vi "Biometry Average Ascan Parameter2String.vi"(8 "error in (no error)":errorcluster caption="错误输入（无错误）", 9 "Biometry Average Standard Deviation":T1, 10 "Biometry Average State":T2, 11 "Biometry Average Parameter":T3) -> (0 "error out":errorcluster caption="错误输出", 2 "Data Output":string[][](array[string]))   [LabVIEW 2015, in "Utility VIs.lvlib"]
doc: "该模板用于创建子VI。"
uses:
  Utility VIs.lvlib
  Database Processing/Support/Table/Biometry Average Parameter.ctl
  Database Processing/Support/Table/Biometry Average State.ctl
  Database Processing/Support/Table/Biometry Average Standard Deviation.ctl
  Database Processing/Database Processing.lvlib
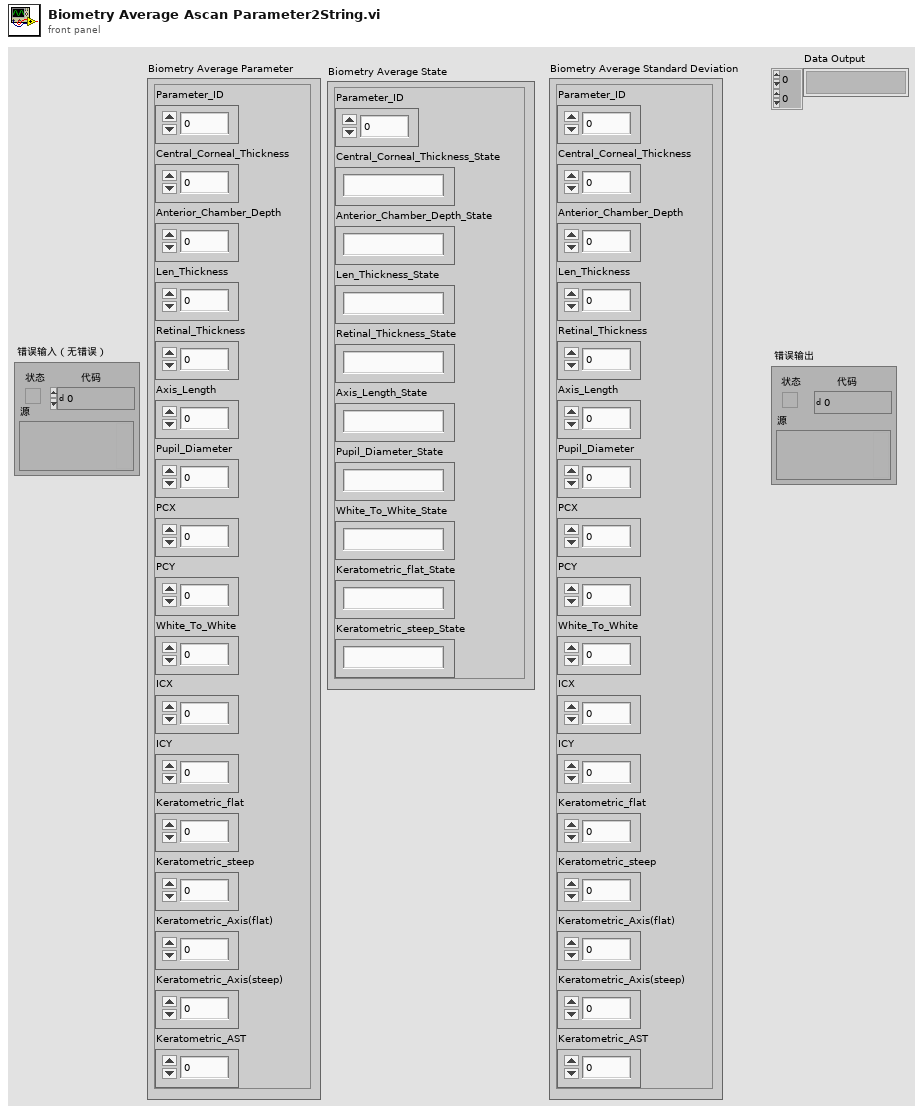
[diagram p1: front panel]
types:
  T1 = typedef "Database Processing.lvlib/Biometry Average Standard Deviation.ctl" = cluster{"Parameter_ID":i64, "Central_Corneal_Thickness":sgl, "Anterior_Chamber_Depth":sgl, "Len_Thickness":sgl, "Retinal_Thickness":sgl, "Axis_Length":sgl, "Pupil_Diameter":sgl, "PCX":sgl, "PCY":sgl, "White_To_White":sgl, "ICX":sgl, "ICY":sgl, "Keratometric_flat":sgl, "Keratometric_steep":sgl, "Keratometric_Axis(flat)":sgl, "Keratometric_Axis(steep)":sgl, "Keratometric_AST":sgl}
  T2 = typedef "Database Processing.lvlib/Biometry Average State.ctl" = cluster{"Parameter_ID":i64, "Central_Corneal_Thickness_State":string, "Anterior_Chamber_Depth_State":string, "Len_Thickness_State":string, "Retinal_Thickness_State":string, "Axis_Length_State":string, "Pupil_Diameter_State":string, "White_To_White_State":string, "Keratometric_flat_State":string, "Keratometric_steep_State":string}
  T3 = typedef "Database Processing.lvlib/Biometry Average Parameter.ctl" = cluster{"Parameter_ID":i64, "Central_Corneal_Thickness":sgl, "Anterior_Chamber_Depth":sgl, "Len_Thickness":sgl, "Retinal_Thickness":sgl, "Axis_Length":sgl, "Pupil_Diameter":sgl, "PCX":sgl, "PCY":sgl, "White_To_White":sgl, "ICX":sgl, "ICY":sgl, "Keratometric_flat":sgl, "Keratometric_steep":sgl, "Keratometric_Axis(flat)":sgl, "Keratometric_Axis(steep)":sgl, "Keratometric_AST":sgl}
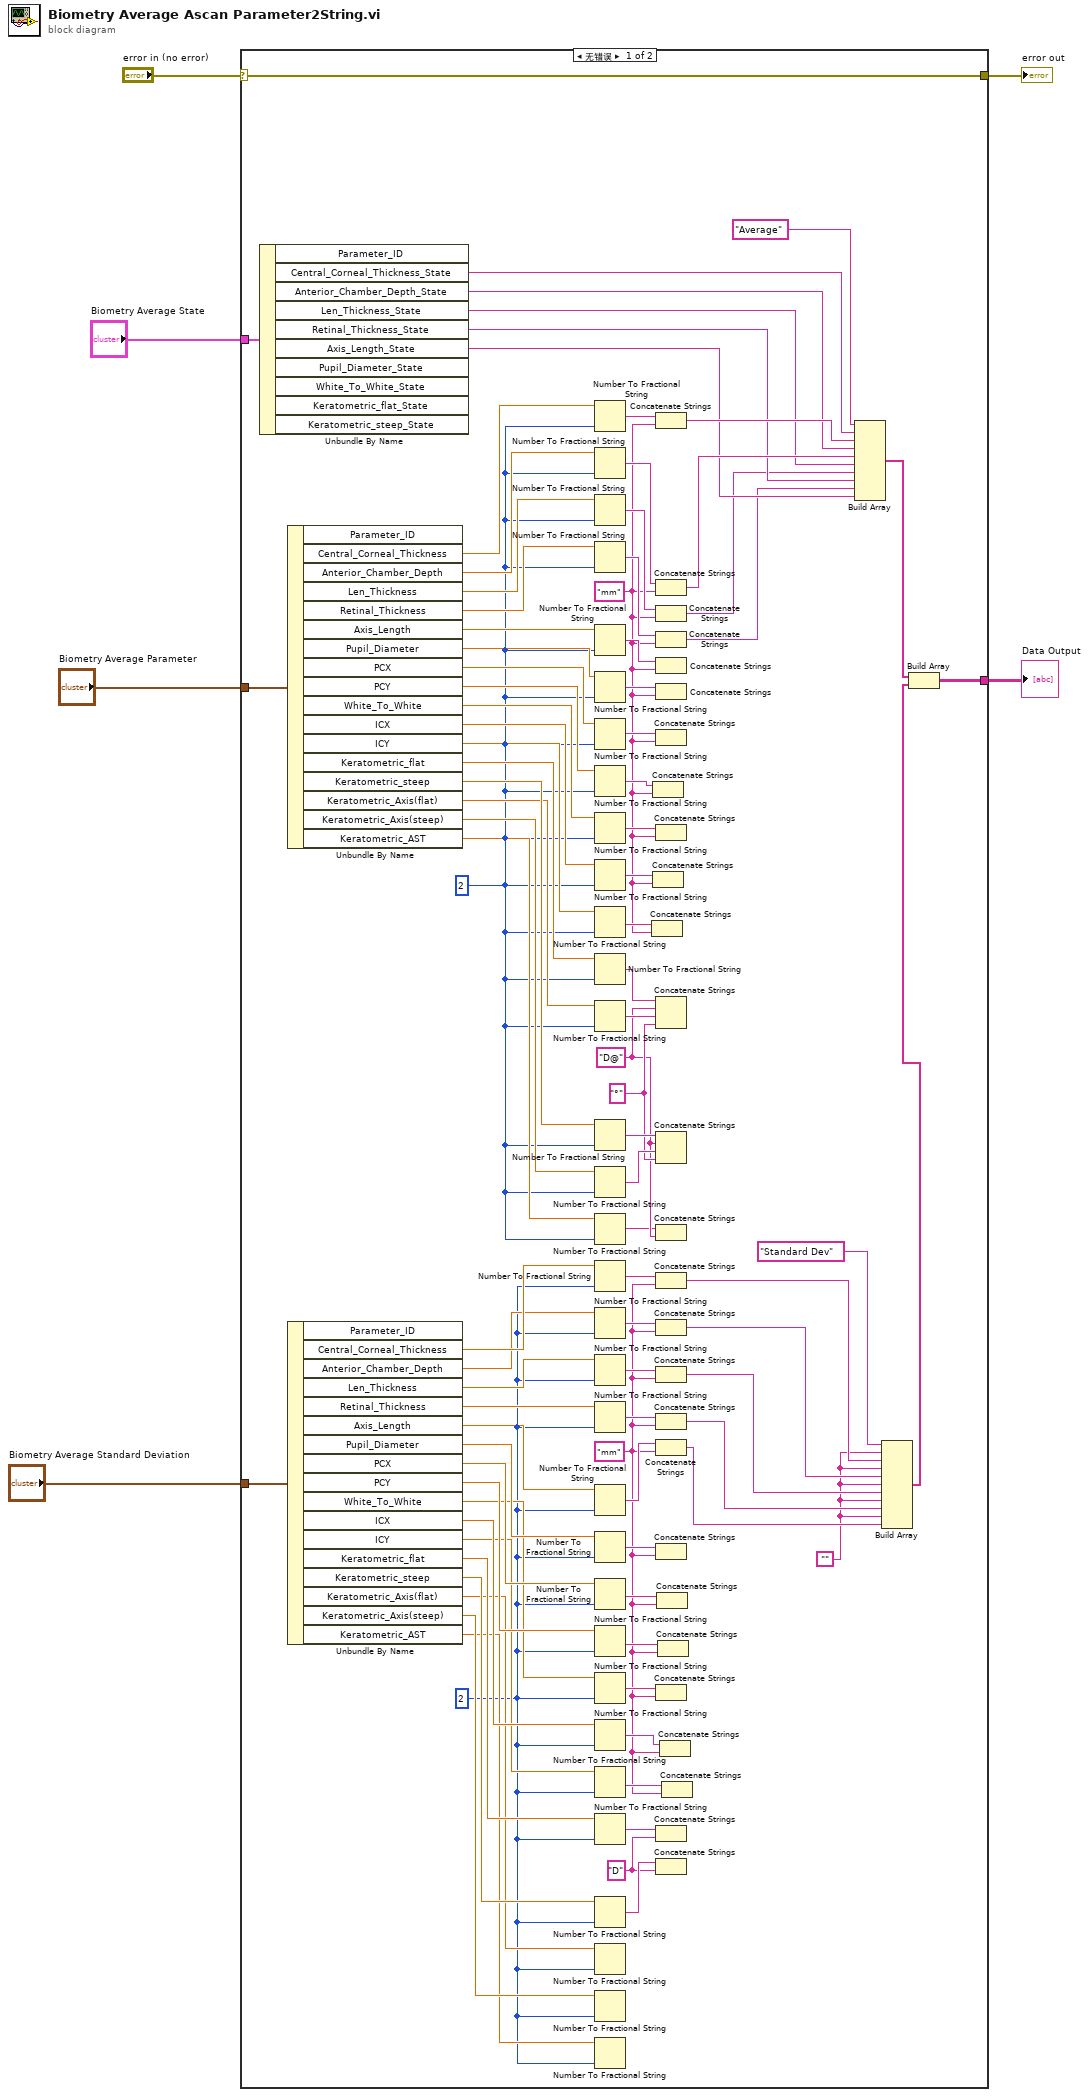
[diagram p0: block diagram]
diagram:
  n1 = case shown="无错误" "error in (no error)" {
    selector: "error in (no error)" -> [w39 w99]
    tunnel: [w39 w99] -> w5
    tunnel: "Biometry Average Parameter" -> [w98 _]
    tunnel: "Biometry Average Standard Deviation" -> [w97 _]
    tunnel: "Biometry Average State" -> [w96 _]
    tunnel: [w9 _] -> w1
    frame No Error {
      w7 = ""
      w40 = "D" ("字符串")
      w27 = "mm" ("字符串")
      w43 = i16 2 ("精度(6)")
      w53 = "°" ("字符串")
      w33 = "D@" ("字符串")
      w34 = "mm" ("字符串")
      w55 = i16 2 ("精度(6)")
      n2 = Unbundle By Name(w96) -> ("Central_Corneal_Thickness_State"=w26:string, "Anterior_Chamber_Depth_State"=w24:string, "Len_Thickness_State"=w22:string, "Retinal_Thickness_State"=w21:string, "Axis_Length_State"=w20:string)  [unwired: 5 out]
      n3 = Unbundle By Name(w98) -> ("Central_Corneal_Thickness"=w95:sgl, "Anterior_Chamber_Depth"=w94:sgl, "Len_Thickness"=w93:sgl, "Retinal_Thickness"=w92:sgl, "Axis_Length"=w91:sgl, "Pupil_Diameter"=w90:sgl, "PCX"=w89:sgl, "PCY"=w88:sgl, "White_To_White"=w87:sgl, "ICX"=w86:sgl, "ICY"=w85:sgl, "Keratometric_flat"=w84:sgl, "Keratometric_steep"=w83:sgl, "Keratometric_Axis(flat)"=w82:sgl, "Keratometric_Axis(steep)"=w57:sgl, "Keratometric_AST"=w56:sgl)  [unwired: 1 out]
      n4 = Unbundle By Name(w97) -> ("Central_Corneal_Thickness"=w81:sgl, "Anterior_Chamber_Depth"=w80:sgl, "Len_Thickness"=w79:sgl, "Retinal_Thickness"=w78:sgl, "Axis_Length"=w77:sgl, "Pupil_Diameter"=w76:sgl, "PCX"=w75:sgl, "PCY"=w74:sgl, "White_To_White"=w73:sgl, "ICX"=w72:sgl, "ICY"=w71:sgl, "Keratometric_flat"=w70:sgl, "Keratometric_steep"=w69:sgl, "Keratometric_Axis(flat)"=w68:sgl, "Keratometric_Axis(steep)"=w45:sgl, "Keratometric_AST"=w44:sgl)  [unwired: 1 out]
      n5 = Number To Fractional String(number=w95, precision (6)=w55) -> (F-format string=w67:string)  [unwired: 2 in]
      n6 = Number To Fractional String(number=w94, precision (6)=w55) -> (F-format string=w66:string)  [unwired: 2 in]
      n7 = Number To Fractional String(number=w93, precision (6)=w55) -> (F-format string=w65:string)  [unwired: 2 in]
      n8 = Number To Fractional String(number=w92, precision (6)=w55) -> (F-format string=w64:string)  [unwired: 2 in]
      n9 = Number To Fractional String(number=w91, precision (6)=w55) -> (F-format string=w63:string)  [unwired: 2 in]
      n10 = Number To Fractional String(number=w90, precision (6)=w55) -> (F-format string=w62:string)  [unwired: 2 in]
      n11 = Number To Fractional String(number=w89, precision (6)=w55) -> (F-format string=w38:string)  [unwired: 2 in]
      n12 = Number To Fractional String(number=w88, precision (6)=w55) -> (F-format string=w37:string)  [unwired: 2 in]
      n13 = Number To Fractional String(number=w87, precision (6)=w55) -> (F-format string=w61:string)  [unwired: 2 in]
      n14 = Number To Fractional String(number=w86, precision (6)=w55) -> (F-format string=w36:string)  [unwired: 2 in]
      n15 = Number To Fractional String(number=w85, precision (6)=w55) -> (F-format string=w35:string)  [unwired: 2 in]
      n16 = Number To Fractional String(number=w84, precision (6)=w55) -> (F-format string=w60:string)  [unwired: 2 in]
      n17 = Number To Fractional String(number=w82, precision (6)=w55) -> (F-format string=w58:string)  [unwired: 2 in]
      n18 = Number To Fractional String(number=w83, precision (6)=w55) -> (F-format string=w59:string)  [unwired: 2 in]
      n19 = Number To Fractional String(number=w57, precision (6)=w55) -> (F-format string=w54:string)  [unwired: 2 in]
      n20 = Number To Fractional String(number=w56, precision (6)=w55) -> (F-format string=w32:string)  [unwired: 2 in]
      n21 = Number To Fractional String(number=w81, precision (6)=w43) -> (F-format string=w52:string)  [unwired: 2 in]
      n22 = Number To Fractional String(number=w80, precision (6)=w43) -> (F-format string=w51:string)  [unwired: 2 in]
      n23 = Number To Fractional String(number=w79, precision (6)=w43) -> (F-format string=w50:string)  [unwired: 2 in]
      n24 = Number To Fractional String(number=w78, precision (6)=w43) -> (F-format string=w49:string)  [unwired: 2 in]
      n25 = Number To Fractional String(number=w77, precision (6)=w43) -> (F-format string=w48:string)  [unwired: 2 in]
      n26 = Number To Fractional String(number=w76, precision (6)=w43) -> (F-format string=w47:string)  [unwired: 2 in]
      n27 = Number To Fractional String(number=w75, precision (6)=w43) -> (F-format string=w31:string)  [unwired: 2 in]
      n28 = Number To Fractional String(number=w74, precision (6)=w43) -> (F-format string=w30:string)  [unwired: 2 in]
      n29 = Number To Fractional String(number=w73, precision (6)=w43) -> (F-format string=w46:string)  [unwired: 2 in]
      n30 = Number To Fractional String(number=w72, precision (6)=w43) -> (F-format string=w29:string)  [unwired: 2 in]
      n31 = Number To Fractional String(number=w71, precision (6)=w43) -> (F-format string=w28:string)  [unwired: 2 in]
      n32 = Number To Fractional String(number=w70, precision (6)=w43) -> (F-format string=w42:string)  [unwired: 2 in]
      n33 = Number To Fractional String(number=w69, precision (6)=w43) -> (F-format string=w41:string)  [unwired: 2 in]
      n34 = Number To Fractional String(number=w68, precision (6)=w43) -> ()  [unwired: 2 in, 1 out]
      n35 = Number To Fractional String(number=w45, precision (6)=w43) -> ()  [unwired: 2 in, 1 out]
      n36 = Number To Fractional String(number=w44, precision (6)=w43) -> ()  [unwired: 2 in, 1 out]
      n37 = Concatenate Strings(w35, w34) -> ()  [unwired: 1 out]
      n38 = Concatenate Strings(w37, w34) -> ()  [unwired: 1 out]
      n39 = Concatenate Strings(w36, w34) -> ()  [unwired: 1 out]
      n40 = Concatenate Strings(w67, w34) -> (w25:string)
      n41 = Concatenate Strings(w66, w34) -> (w23:string)
      n42 = Concatenate Strings(w65, w34) -> (w19:string)
      n43 = Concatenate Strings(w64, w34) -> (w18:string)
      n44 = Concatenate Strings(w63, w34) -> ()  [unwired: 1 out]
      n45 = Concatenate Strings(w62, w34) -> ()  [unwired: 1 out]
      n46 = Concatenate Strings(w38, w34) -> ()  [unwired: 1 out]
      n47 = Concatenate Strings(w61, w34) -> ()  [unwired: 1 out]
      n48 = Concatenate Strings(w60, w33, w58, w53) -> ()  [unwired: 1 out]
      n49 = Concatenate Strings(w59, w33, w54, w53) -> ()  [unwired: 1 out]
      n50 = Concatenate Strings(w32, w33) -> ()  [unwired: 1 out]
      n51 = Concatenate Strings(w52, w27) -> (w17:string)
      n52 = Concatenate Strings(w51, w27) -> (w16:string)
      n53 = Concatenate Strings(w50, w27) -> (w15:string)
      n54 = Concatenate Strings(w49, w27) -> (w14:string)
      n55 = Concatenate Strings(w48, w27) -> (w13:string)
      n56 = Concatenate Strings(w47, w27) -> ()  [unwired: 1 out]
      n57 = Concatenate Strings(w46, w27) -> ()  [unwired: 1 out]
      n58 = Concatenate Strings(w42, w40) -> ()  [unwired: 1 out]
      n59 = Concatenate Strings(w41, w40) -> ()  [unwired: 1 out]
      n60 = Concatenate Strings(w31, w27) -> ()  [unwired: 1 out]
      n61 = Concatenate Strings(w30, w27) -> ()  [unwired: 1 out]
      n62 = Concatenate Strings(w29, w27) -> ()  [unwired: 1 out]
      n63 = Concatenate Strings(w28, w27) -> ()  [unwired: 1 out]
      n64 = Build Array("Average" ("元素"), w26, w25, w24, w23, w22, w19, w21, w18, w20) -> (w11:string[])
      n65 = Build Array("Standard Dev" ("元素"), w7, w17, w7, w16, w7, w15, w7, w14, w7, w13) -> (w10:string[])
      n66 = Build Array(w11, w10) -> (w9:string[][])
    }
    frame Error {
    }
  }
  "error out" <- w5
  "Data Output" <- w1
